vi "CameraControler Analyze.vi"(9 "Climbing Manual Enabled":bool, 11 "JoystickDevRef":T1) -> (1 "axis 3 (rotation)":dbl, 2 "Y":dbl, 3 "Flipper Override":bool, 4 "stop auto camera movement":bool, 5 "Center on Target":bool, 7 "View Ground":bool)   [LabVIEW 2012]
uses:
  <vilib>/Rock Robotics/WPI/Joystick/WPI_JoystickDevRef.ctl
  <vilib>/Rock Robotics/WPI/Joystick/WPI_JoystickDeviceEnum.ctl
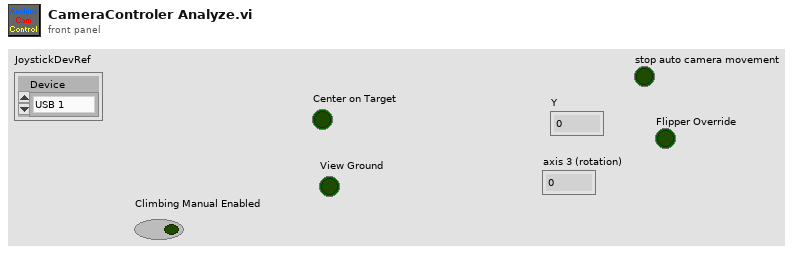
[diagram p1: front panel]
types:
  T1 = typedef "WPI_JoystickDevRef.ctl" = cluster{"Device":T2}
  T2 = typedef "WPI_JoystickDeviceEnum.ctl" = enum16{"USB 1", "USB 2", "USB 3", "USB 4", "Kinect 1", "Kinect 2"}
  T3 = typedef "WPI_JoystickButtonState.ctl" = cluster{"Button 1":bool, "Button 2":bool, "Button 3":bool, "Button 4":bool, "Button 5":bool, "Button 6":bool, "Button 7":bool, "Button 8":bool, "Button 9":bool, "Button 10":bool, "Button 11":bool, "Button 12":bool}
  T4 = cluster{"axis 1 (x)":dbl, "axis 2 (y)":dbl, "axis 3 (throttle)":dbl, "axis 4":dbl, "axis 5":dbl, "axis 6":dbl}
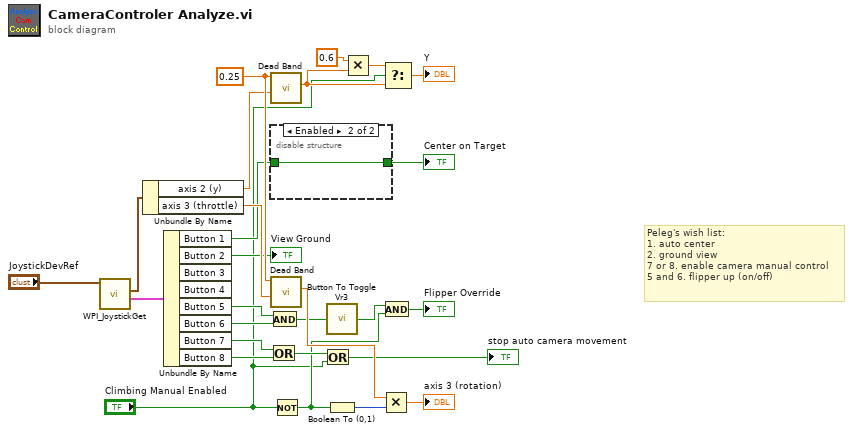
[diagram p0: block diagram]
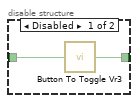
[diagram p2: hidden frame]
diagram:
  w23 = 0.25 ("Dead Band")
  # "Peleg's wish list:\n1. auto center\n2. ground view\n7 or 8. enable camera manual control\n5 and 6. flipper up (on/off)"
  n1 = call <vilib>:"WPI_JoystickGet.vi"("JoystickDevRef"="JoystickDevRef") -> ("Buttons"=w25:T3, "Axes"=w26:T4)  [unwired: 4 in, 1 out]
  n2 = Unbundle By Name(w26) -> ("axis 2 (y)"=w22:dbl, "axis 3 (throttle)"=w24:dbl)
  n3 = Unbundle By Name(w25) -> ("Button 1"=w12:bool, "Button 2"=→"View Ground":bool, "Button 5"=w19:bool, "Button 6"=w18:bool, "Button 7"=w14:bool, "Button 8"=w15:bool)  [unwired: 2 out]
  n4 = Or(x=w14, y=w15) -> (x .or. y?=w11:bool)
  n5 = And(x=w19, y=w18) -> (x .and. y?=w17:bool)
  n6 = call "Dead Band.vi"("Axis In"=w22, "Dead Band"=w23) -> ("Axis Out"=w3:dbl)  [unwired: 9 in]
  n7 = disable-structure shown="Enabled" {
    disable-tunnel: [w29 w30] -> w13
    disable-tunnel: w12 -> [w28 w30]
    frame Disabled {
      n8 = call "Button To Toggle Vr3.vi"("InValue"=w28) -> ("Result"=w29:bool)
    }
    frame Enabled {
    }
  }
  "Center on Target" <- w13
  n9 = call "Dead Band.vi"("Axis In"=w24, "Dead Band"=w23) -> ("Axis Out"=w20:dbl)  [unwired: 9 in]
  n10 = Not(x="Climbing Manual Enabled") -> (.not. x?=w8:bool)
  n11 = Or(x=w11, y="Climbing Manual Enabled") -> (x .or. y?=→"stop auto camera movement":bool)
  n12 = call "Button To Toggle Vr3.vi"("InValue"=w17) -> ("Result"=w16:bool)
  n13 = Boolean To (0,1)(Boolean=w8) -> (0, 1=w6:i16)
  n14 = Multiply(x=0.6, y=w3) -> (x*y=w2:dbl)
  n15 = Multiply(x=w20, y=w6) -> (x*y=→"axis 3 (rotation)":dbl)
  n16 = And(x=w16, y=w8) -> (x .and. y?=→"Flipper Override":bool)
  n17 = Select(t=w2, s="Climbing Manual Enabled", f=w3) -> (s? t:f=→"Y":dbl)
